vi "Relabel Annotation.vi"(8 "error in (no error)":errorcluster, 9 "New Name":string, 10 "Old Name":string, 11 "FSM.Edge in":refnum<class "FSM.Edge.lvclass">) -> (0 "error out":errorcluster, 3 "FSM.Edge out":refnum<class "FSM.Edge.lvclass">)   [LabVIEW 2015, in "FSM.Edge.lvclass"]
uses:
  FSM.Edge.lvclass
  FSM.Edge.lvclass/FSM.Edge.ctl
  FSM.Annotation/FSM.Annotation.lvclass/FSM.Annotation.ctl
  FSM.Annotation/Read Items.vi
  FSM.Annotation/Write Items.vi
  FSM.Annotation/FSM.Annotation.lvclass
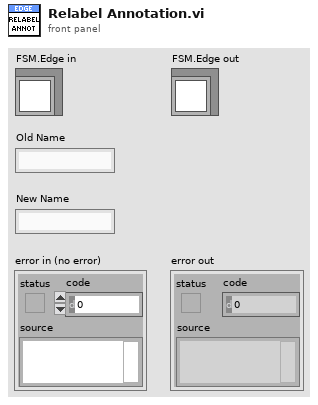
[diagram p1: front panel]
types:
  T1 = cluster{"Name":string, "Style":enum16{"Plain", "On", "Off", "On-Off"}}[]
  T2 = cluster{"Name":string, "Style":enum16{"Plain", "On", "Off", "On-Off"}}
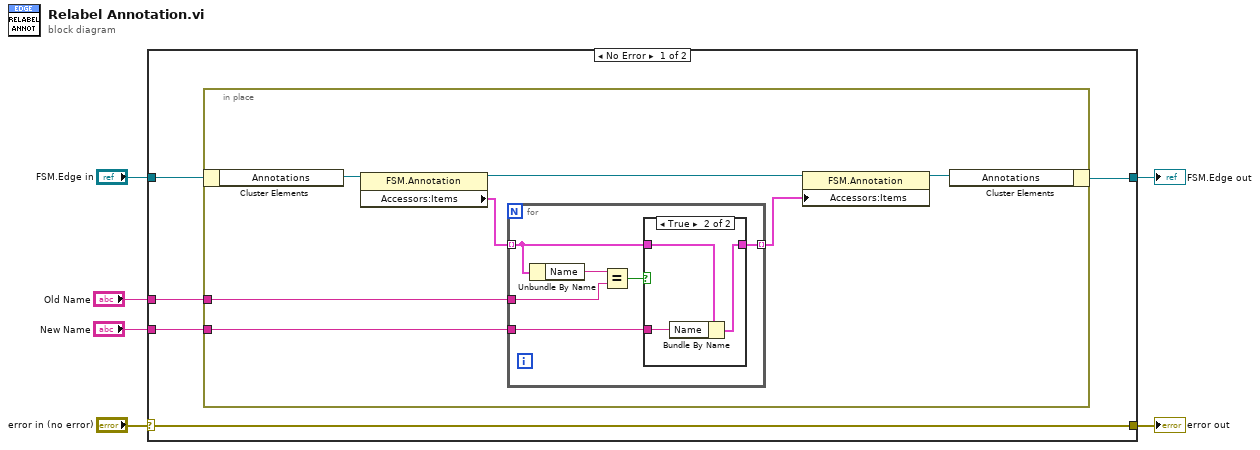
[diagram p0: block diagram]
diagram:
  n1 = case shown="No Error" "error in (no error)" {
    selector: "error in (no error)" -> [w11 w30]
    tunnel: [w11 w30] -> w5
    tunnel: [w7 w29] -> w3
    tunnel: "FSM.Edge in" -> [w10 w29]
    tunnel: "Old Name" -> [w9 _]
    tunnel: "New Name" -> [w8 _]
    frame No Error {
      n2 = in-place {
        in-place-border: w9 -> [w16]
        in-place-border: w8 -> [w13]
        n3 = in-place-cluster #1(w10) -> ("Annotations"=w18:refnum<class "FSM.Annotation.lvclass">)
        n4 = property class="FSM.Annotation"(reference=w18) -> (reference out=w14:refnum<class "FSM.Annotation.lvclass">, "Accessors:Items"=w17:T1)  [unwired: 1 in, 1 out]
        n5 = for {
          tunnel: w17 -> [w21] mode=indexing
          tunnel: w16 -> [w23]
          tunnel: [w20] -> w12 mode=indexing
          tunnel: w13 -> [w19]
          n6 = Unbundle By Name(w21) -> ("Name"=w24:string)
          n7 = Equal?(x=w24, y=w23) -> (x = y?=w22:bool)
          n8 = case shown="True" w22 {
            tunnel: w21 -> [w25 w28]
            tunnel: [w25 w27] -> w20
            tunnel: w19 -> [_ w26]
            frame False {
            }
            frame True {
              n9 = Bundle By Name(cluster=w28, "Name"=w26) -> (w27:T2)
            }
          }
        }
        n10 = property class="FSM.Annotation"(reference=w14, "Accessors:Items"=w12) -> (reference out=w15:refnum<class "FSM.Annotation.lvclass">)  [unwired: 1 in, 1 out]
        n11 = in-place-cluster #1("Annotations"=w15) -> (w7:refnum<class "FSM.Edge.lvclass">)
      }
    }
    frame Error {
    }
  }
  "error out" <- w5
  "FSM.Edge out" <- w3
